vi "StatusSendStatEnb.vi"(9 "StatReplies":T1={"DecodeMode"="Stat", "LastSerial"=0, "StatReset"=FALSE, "StatCmd"="", "StatCmdReply"="", "StatCmdReplySerial"=0, "StatusPrefix"="", "StatusData"="", "CmdArray"=[0, 2, 1, 4, 16, 230, 2, 1, 0], "SendOut"=FALSE, "StringCmd"=FALSE, "CmdString1"="", "CmdString0"="", "Astring1"=FALSE, "ManCmd"=""}, 10 "CmdData":string, 11 "error":errorcluster) -> (3 "EnableOut":bool)   [LabVIEW 2019]
uses:
  TypeDefinitions/StatTcpRelies.ctl
  Main/NmlTypeDefinitions/230.0-JointMode.ctl
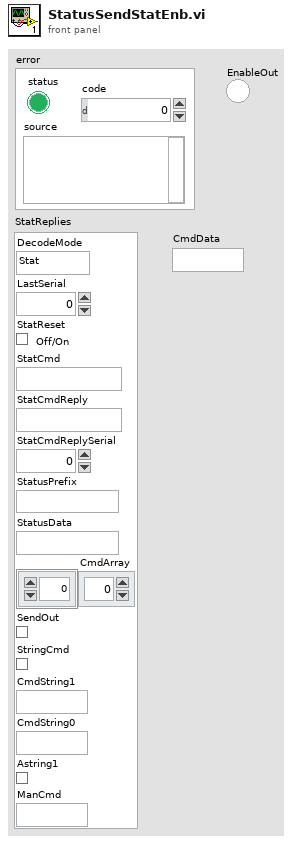
[diagram p1: front panel]
types:
  T1 = typedef "StatTcpRelies.ctl" = cluster{"DecodeMode":string, "LastSerial":u32, "StatReset":bool, "StatCmd":string, "StatCmdReply":string, "StatCmdReplySerial":u32, "StatusPrefix":string, "StatusData":string, "CmdArray":T2, "SendOut":bool, "StringCmd":bool, "CmdString1":string, "CmdString0":string, "Astring1":bool, "ManCmd":string}
  T2 = typedef "230.0-JointMode.ctl" = u32[]
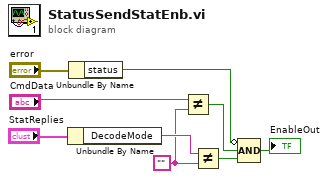
[diagram p0: block diagram]
diagram:
  w2 = ""
  n1 = Unbundle By Name("StatReplies") -> ("DecodeMode"=w7:string)
  n2 = Unbundle By Name("error") -> ("status"=w9:bool)
  n3 = Not Equal?(x="CmdData", y=w2) -> (x != y?=w1:bool)
  n4 = Not Equal?(x=w7, y=w2) -> (x != y?=w8:bool)
  n5 = Compound Arithmetic op=AND(invert w9, w1, w8) -> (→"EnableOut":bool)
